vi "Get Default TSA Report Path.vi"(8 "error in (no error)":errorcluster, 11 "TestStand Sequence Analyzer Project":path) -> (0 "error out":errorcluster, 3 "TSA Report Path":path)   [LabVIEW 2014, in "SLL TestStand.lvlib"]
doc: "Generates the default TSA Report Path based on the TSA Project Name.\n\n<Temp Directory>/<TSA Project Name>.xml"
uses:
  SLL TestStand.lvlib
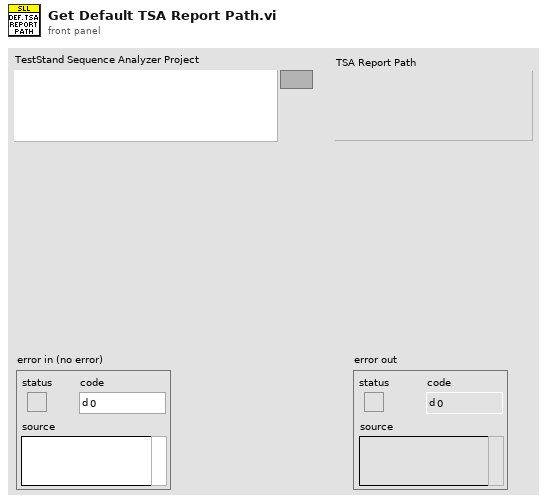
[diagram p1: front panel]
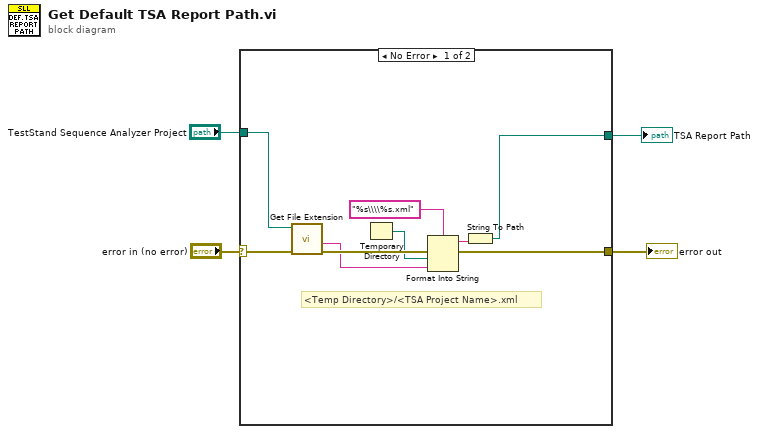
[diagram p0: block diagram]
diagram:
  n1 = case shown="No Error" "error in (no error)" {
    selector: "error in (no error)" -> [w13 w14]
    tunnel: [w10 w14] -> w3
    tunnel: "TestStand Sequence Analyzer Project" -> [w11 _]
    tunnel: [w5 _] -> w1
    frame No Error {
      # "<Temp Directory>/<TSA Project Name>.xml"
      n2 = call <vilib>:"Get File Extension.vi"("error in (no error)"=w13, "file"=w11) -> ("error out"=w12:errorcluster, "filename without extension"=w7:string)  [unwired: 6 in, 2 out]
      n3 = Temporary Directory() -> (w8:path)
      n4 = Format Into String(format string="%s\\\\%s.xml", error in=w12, w8, w7) -> (resulting string=w6:string, error out=w10:errorcluster)  [unwired: 1 in]
      n5 = String To Path(string=w6) -> (path=w5:path)
    }
    frame Error {
    }
  }
  "error out" <- w3
  "TSA Report Path" <- w1
